vi "PS long Name to Short.vi"(11 "String":string) -> (3 "whole match":string)   [LabVIEW 2020]
uses:
  <vilib>/regexp/Match Regular Expression.xnode
panel:
  # "\"Pretreatment settings (PS)\""
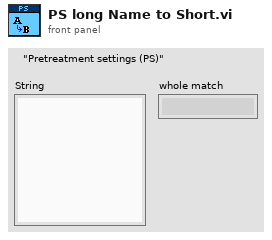
[diagram p1: front panel]
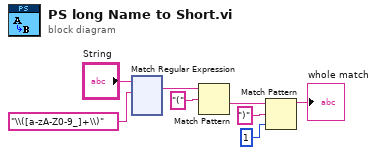
[diagram p0: block diagram]
diagram:
  n1 = xnode "Match Regular Expression"("input string"="String", "regular expression"="\\([a-zA-Z0-9_]+\\)") -> ("whole match"=w4:string)  [unwired: 4 in, 4 out]
  n2 = Match Pattern(string=w4, regular expression="(") -> (after substring=w6:string)  [unwired: 1 in, 3 out]
  n3 = Match Pattern(string=w6, regular expression=")", offset (0)=1) -> (before substring=→"whole match":string)  [unwired: 3 out]
